vi "onListRequirements.vi"(8 "error in (no error)":errorcluster, 10 "Filter":T1, 11 "Pips in":refnum<class "Pips.lvclass">) -> (0 "error out":errorcluster, 2 "RequirementIDs":string[](array[string]), 3 "Pips out":refnum<class "Pips.lvclass">)   [LabVIEW 2021, in "Bananas.lvlib" / "Pips.lvclass"]
uses:
  Pips.lvclass
  pip_filter -- enum.ctl
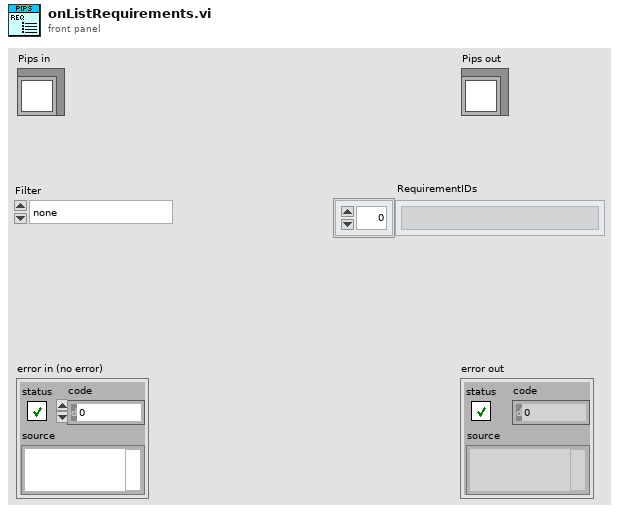
[diagram p1: front panel]
types:
  T1 = typedef "Bananas.lvlib/Pips.lvclass/pip_filter -- enum.ctl" = enum16{"none", "passed", "skipped", "covered", "uncovered"}
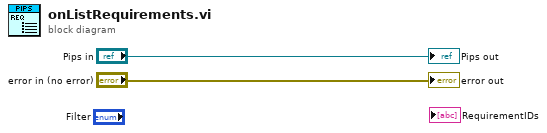
[diagram p0: block diagram]
diagram:
  "error out" <- "error in (no error)"
  "Pips out" <- "Pips in"
